vi "Plot Type Read.vi"(4 "error in (no error)":errorcluster, 6 "Container State":T9, 7 "Display State In":T1={"GPR Graph Info"={"Display Type"=enum."Intensity Plot", "Display Info"={"X Scale"={"X Scale Label"=TRUE, "X Scale Name"="Trace #", "X Scale Visible"=TRUE, "dx"=1.0}, "Y Scale"={"X Scale Label"=TRUE, "X Scale Name"="Time (s)", "X Scale Visible"=TRUE, "dt"=4e-10}, "BackGround Color"=16448250}, "Trace Options"={"Trace Amplitude"=1.0, "Trace Color"=0, "Fill options"=enum."No Fill"}, "Intensity Options"={"Color Scale"=enum."RWB"}}, "Transpose Data"=FALSE, "Run-time Edit"=FALSE, "Clear Request"=FALSE}) -> (0 "error out":errorcluster, 2 "Value":T3, 3 "Display State Out":T1={"GPR Graph Info"={"Display Type"=enum."Intensity Plot", "Display Info"={"X Scale"={"X Scale Label"=TRUE, "X Scale Name"="Trace #", "X Scale Visible"=TRUE, "dx"=1.0}, "Y Scale"={"X Scale Label"=TRUE, "X Scale Name"="Time (s)", "X Scale Visible"=TRUE, "dt"=4e-10}, "BackGround Color"=16448250}, "Trace Options"={"Trace Amplitude"=1.0, "Trace Color"=0, "Fill options"=enum."No Fill"}, "Intensity Options"={"Color Scale"=enum."RWB"}}, "Transpose Data"=FALSE, "Run-time Edit"=FALSE, "Clear Request"=FALSE})   [LabVIEW 2009, in "GPR.xctl"]
uses:
  GPR.xctl
  <vilib>/_xctls/Container State.ctl
  Controls/Display Types.ctl
  Abilities/GPR State.ctl
  Controls/GPR Graph Info.ctl
  Controls/Display Info.ctl
  Controls/Trace Options.ctl
  Controls/Fill Options.ctl
  Controls/Intensity Options.ctl
  Controls/Color Scales.ctl
  <vilib>/_xctls/XControlSupport.lvlib
panel:
  # "Replace the Value Indicator below with an Indicator of desired type.\nDo not remove this Indicator or the others from the connector pane. \nDo not change the connector pane pattern.\nThe Value Indicator should always be the second terminal from top on the output side in the connector pane."
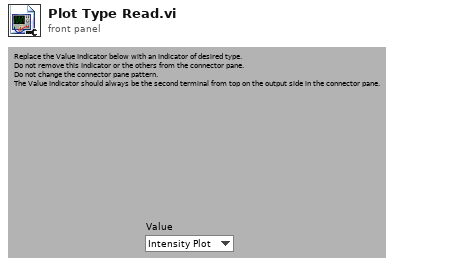
[diagram p1: front panel]
types:
  T1 = typedef "GPR.xctl/GPR State.ctl" = cluster{"GPR Graph Info":T2, "Transpose Data":bool, "Run-time Edit":bool, "Clear Request":bool}
  T2 = typedef "GPR Graph Info.ctl" = cluster{"Display Type":T3, "Display Info":T4, "Trace Options":T5, "Intensity Options":T7}
  T3 = typedef "Display Types.ctl" = enum16{"Intensity Plot", "Wiggle Trace"}
  T4 = typedef "Display Info.ctl" = cluster{"X Scale":cluster{"X Scale Label":bool, "X Scale Name":string, "X Scale Visible":bool, "dx":dbl}, "Y Scale":cluster{"X Scale Label":bool, "X Scale Name":string, "X Scale Visible":bool, "dt":dbl}, "BackGround Color":u32}
  T5 = typedef "Trace Options.ctl" = cluster{"Trace Amplitude":dbl, "Trace Color":u32, "Fill options":T6}
  T6 = typedef "Fill Options.ctl" = enum32{"No Fill", "Fill Positive", "Fill Negative"}
  T7 = typedef "Intensity Options.ctl" = cluster{"Color Scale":T8}
  T8 = typedef "Color Scales.ctl" = enum16{"RGB", "RWB", "BGR", "BWR", "BW", "WB"}
  T9 = typedef "XControlSupport.lvlib/Container State.ctl" = cluster{"Indicator?":bool, "Run Mode?":bool, " Refnum":refnum<vi>}
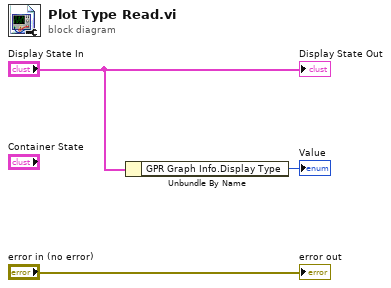
[diagram p0: block diagram]
diagram:
  n1 = Unbundle By Name("Display State In") -> ("GPR Graph Info.Display Type"=→"Value":T3)
  "error out" <- "error in (no error)"
  "Display State Out" <- "Display State In"
